vi "GetKeyState.vi"(10 "Virtual Keys":i32(ring)=20 format="%02x" items=["Not used", "Left mouse button", "Right mouse button", "Control-break processing", "Middle mouse button (three-button mouse)", "X1 mouse button", "X2 mouse button", "0x07 - Undefined", "BACKSPACE key", "TAB key", "0x0A Reserved", "0x0B Reserved", "CLEAR key", "ENTER key", "0x0E Undefined", "0x0F Undefined", "SHIFT key", "CTRL key", "ALT key", "PAUSE key", "CAPS LOCK key", "IME Hangul mode", "0x16 Undefined", "IME Junja mode", "IME final mode", "IME Hanja mode", "0x1A Undefined", "ESC key", "IME convert", "IME nonconvert", "IME accept", "IME mode change request", "SPACEBAR", "PAGE UP key", "PAGE DOWN key", "END key", "HOME key", "LEFT ARROW key", "UP ARROW key", "RIGHT ARROW key", "DOWN ARROW key", "SELECT key", "PRINT key", "EXECUTE key", "PRINT SCREEN key", "INS key", "DEL key", "HELP key", "0 key", "1 key", "2 key", "3 key", "4 key", "5 key", "6 key", "7 key", "8 key", "9 key", "0x3A Undefined", "0x3B Undefined", "0x3C Undefined", "0x3D Undefined", "0x3E Undefined", "0x3F Undefined", "0x40 Undefined", "A key", "B key", "C key", "D key", "E key", "F key", "G key", "H key", "I key", "J key", "K key", "L key", "M key", "N key", "O key", "P key", "Q key", "R key", "S key", "T key", "U key", "V key", "W key", "X key", "Y key", "Z key", "Left Windows key (Natural Keyboard)", "Right Windows key (Natural keyboard)", "Applications key (Natural keyboard)", "Reserved", "Computer Sleep key", "Numeric keypad 0 key", "Numeric keypad 1 key", "Numeric keypad 2 key", "Numeric keypad 3 key", "Numeric keypad 4 key", "Numeric keypad 5 key", "Numeric keypad 6 key", "Numeric keypad 7 key", "Numeric keypad 8 key", "Numeric keypad 9 key", "Multiply key", "Add key", "Separator key", "Substract key", "Decimal key", "Divide key", "F1 key", "F2 key", "F3 key", "F4 key", "F5 key", "F6 key", "F7 key", "F8 key", "F9 key", "F10 key", "F11 key", "F12 key", "F13 key", "F14 key", "F15 key", "F16 key", "F17 key", "F18 key", "F19 key", "F20 key", "F21 key", "F22 key", "F23 key", "F24 key", "0x88 Unassigned", "0x89 Unassigned", "0x8A Unassigned", "0x8B Unassigned", "0x8C Unassigned", "0x8D Unassigned", "0x8E Unassigned", "0x8F Unassigned", "NUM LOCK key", "SCROLL LOCK key", "0x92 OEM specific", "0x93 OEM specific", "0x94 OEM specific", "0x95 OEM specific", "0x96 OEM specific", "0x97 Unassigned", "0x98 Unassigned", "0x99 Unassigned", "0x9A Unassigned", "0x9B Unassigned", "0x9C Unassigned", "0x9D Unassigned", "0x9E Unassigned", "0x9F Unassigned", "Lefth SHIFT key", "Right SHIFT key", "Left CONTROL key", "Right CONTROL key", "Left MENU key", "Right MENU key", "Browser Back key", "Browser Forward key", "Browser Refresh key", "Browser Stop key", "Browser Search key", "Browser Favorites key", "Browser Start and Home key", "Volume Mute key", "Volume Down key", "Volume Up key", "Next Track key", "Previous Track key", "Stop Media key", "Play/Pause Media key", "Start Mail key", "Select Media key", "Start Application 1 key", "Start Application 2 key", "0xB8 Reserved", "0xB9 Reserved", "US standard keyboard \" ;:' key"]) -> (2 "Key State":bool)   [LabVIEW 2009]
doc: "This VI get the key state using the user32.dll GetKeyState API\n\n<b>Inputs</b>\nVirtual key: Select the virtual key to be queried\n\n<b>Outputs</b>\nKey State: Indicates if the virtual key is enabled(True) / Disabled (False)\n\n<b>Extra information </b>\nLibrary name: User32.dll\nFunction name: GetKeyState\nPrototype: int16 GetKeyState(int32 nVirtualKey);\n\nDeveloped by eZ\nAug 17th 2010"
uses:
  user32.dll
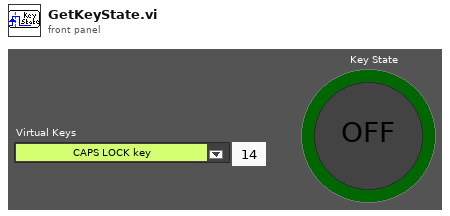
[diagram p1: front panel]
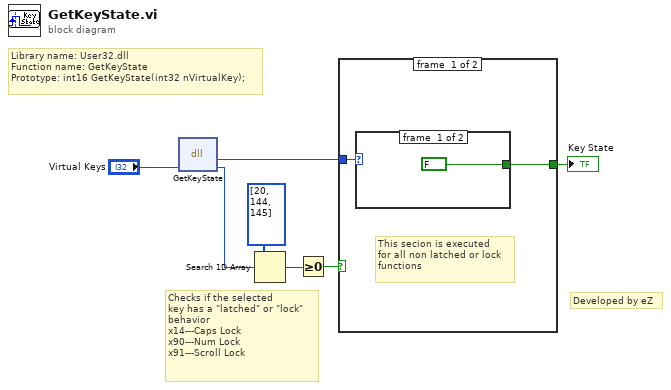
[diagram p0: block diagram]
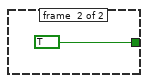
[diagram p2: hidden frame]
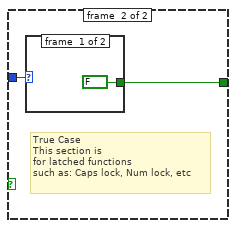
[diagram p3: hidden frame]
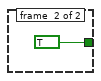
[diagram p4: hidden frame]
diagram:
  # "Developed by eZ"
  # "Checks if the selected\nkey has a \"latched\" or \"lock\"\nbehavior\nx14---Caps Lock\nx90---Num Lock\nx91---Scroll Lock"
  # "Library name: User32.dll\nFunction name: GetKeyState\nPrototype: int16 GetKeyState(int32 nVirtualKey);"
  n1 = dll-call lib="user32.dll" fn="GetKeyState"("Virtual Key"="Virtual Keys") -> ("return type"=w2:i16, "Virtual Key"=w6:i32)  [unwired: 3 in, 2 out]
  n2 = Search 1D Array(1D array=i32[] [20, 144, 145], element=w6) -> (index of element=w4:i32)  [unwired: 1 in]
  n3 = Greater Or Equal To 0?(x=w4) -> (x >= 0?=w3:bool)
  n4 = case shown="False" w3 {
    tunnel: w2 -> [w8 w13]
    tunnel: [w9 w12] -> w1
    frame #0 {
      # "This secion is executed\nfor all non latched or lock\nfunctions"
      n5 = case shown="-128, -127" w8 {
        tunnel: [FALSE TRUE] -> w9
        frame #0 {
        }
        frame #1 {
        }
      }
    }
    frame #1 {
      # "True Case\nThis section is\nfor latched functions\nsuch as: Caps lock, Num lock, etc"
      n6 = case shown="-127, 1" w13 {
        tunnel: [FALSE TRUE] -> w12
        frame #0 {
        }
        frame #1 {
        }
      }
    }
  }
  "Key State" <- w1
